vi "Coherent Fault FP String.vi"(11 "I/p String":string) -> (3 "O/P String":string)   [LabVIEW 2020]
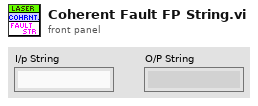
[diagram p1: front panel]
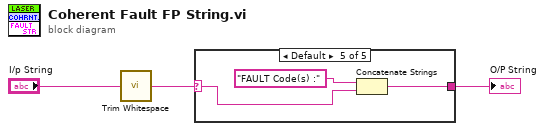
[diagram p0: block diagram]
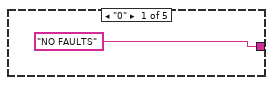
[diagram p2: hidden frame]
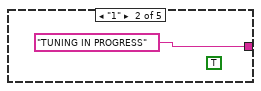
[diagram p3: hidden frame]
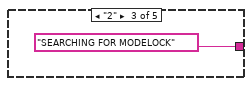
[diagram p4: hidden frame]
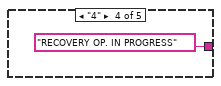
[diagram p5: hidden frame]
diagram:
  n1 = call <vilib>:"Trim Whitespace.vi"("string"="I/p String") -> ("trimmed string"=w2:string)  [unwired: 1 in]
  n2 = case shown="Default" w2 {
    selector: w2 -> [_ _ _ _ w9]
    tunnel: ["NO FAULTS" "TUNING IN PROGRESS" "SEARCHING FOR MODELOCK" "RECOVERY OP. IN PROGRESS" w8] -> w3
    frame "0" {
    }
    frame "1" {
      (unwired) TRUE
    }
    frame "2" {
    }
    frame "4" {
    }
    frame Default {
      n3 = Concatenate Strings("FAULT Code(s) :", w9) -> (w8:string)
    }
  }
  "O/P String" <- w3
